vi "Data Folder.vi"(8 "error in (no error)":errorcluster, 11 "Node Ptr":T2 format="%.0x") -> (0 "error out":errorcluster)   [LabVIEW 2020, in "RefMem DMA System Explorer.lvlib"]
uses:
  RefMem DMA System Explorer.lvlib
  <vilib>/NI VeriStand/Custom Device API/Custom Device Item Ref.ctl
  controls/Data Channel Type.ctl
  <vilib>/NI VeriStand/Custom Device API/Custom Device Channel.ctl
  <vilib>/NI VeriStand/Custom Device API/Custom Device Channel Type.ctl
  Shared/Constants.vi
  <vilib>/NI VeriStand/Custom Device API/Get Item Property (U16).vi
  <vilib>/NI VeriStand/Custom Device API/Get Item Property (U32).vi
  <vilib>/NI VeriStand/Custom Device Tools/Custom Device Utility Library/NI VeriStand - Search for Item by Name.vi
  <vilib>/NI VeriStand/Custom Device API/NI VeriStand - Find next valid Label.vi
  <vilib>/NI VeriStand/Custom Device API/Set Item Property (U16).vi
  <vilib>/NI VeriStand/Custom Device API/Set Item Property (U32).vi
  <vilib>/NI VeriStand/Custom Device API/Custom Device API.lvlib
  Shared/RefMem DMA Shared.lvlib
  <vilib>/NI VeriStand/Custom Device Tools/Custom Device Utility Library/Custom Device Utility Library.lvlib
panel:
  in  "Type":T1
  in  "Block Address":u32
  in  "Add Data Channel":bool
  in  "Header":cluster{"Section Name":string}={"Section Name"="Data Folder"}
  in  "Description":string
  in  "Name":string
  # "In channels (doubles)"
  # "Channels to write has to be in row\nChannels to read can have space in between"
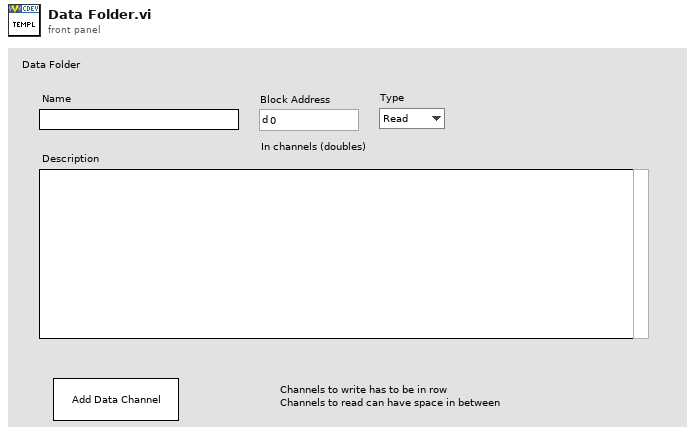
[diagram p1: front panel]
types:
  T1 = typedef "RefMem DMA System Explorer.lvlib/Data Channel Type.ctl" = enum16{"Read", "Write"}
  T2 = typedef "Custom Device API.lvlib/Custom Device Item Ref.ctl" = u64
  T3 = typedef "Custom Device API.lvlib/Custom Device Item Info.ctl" = cluster{"Name":string, "Is Channel":bool, "GUID":string, "Is Waveform":bool}
  T4 = typedef "Custom Device API.lvlib/Custom Device Channel.ctl" = cluster{"Type":T5, "Units":string, "Default Value":dbl, "Faultable":bool, "Scalable":bool}
  T5 = typedef "Custom Device API.lvlib/Custom Device Channel Type.ctl" = enum16{"Input", "Output"}
  T6 = typedef "Custom Device API.lvlib/Custom Device Commands.ctl" = enum16{"Default", "Item renamed", "Shutdown", "Dynamic button pressed"}
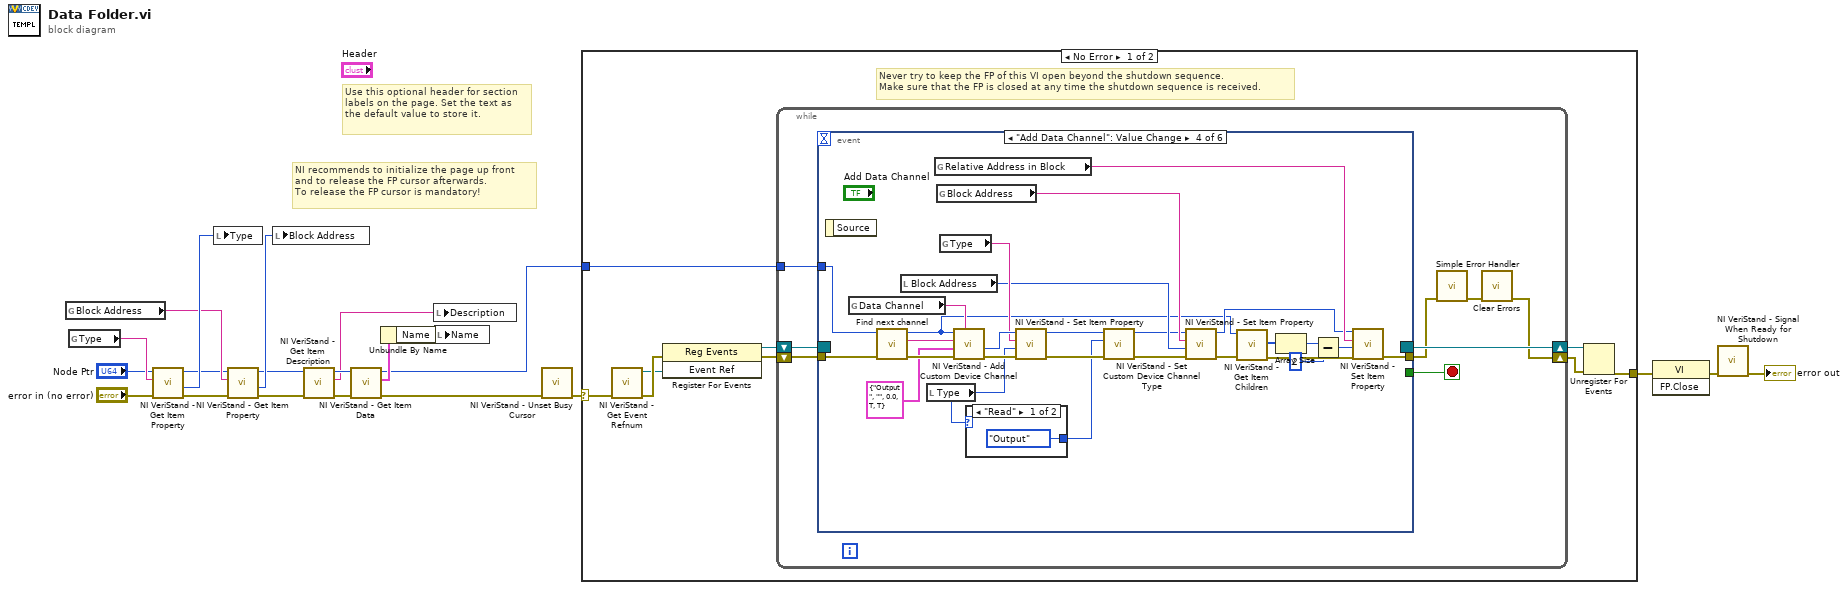
[diagram p0: block diagram]
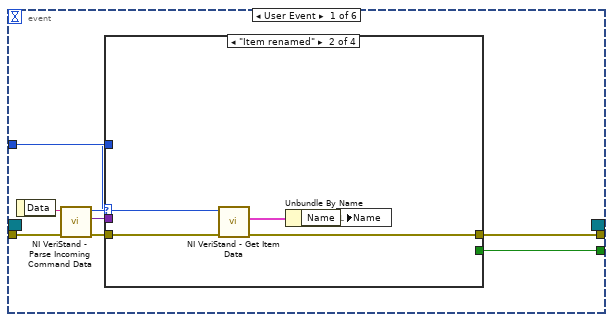
[diagram p2: hidden frame]
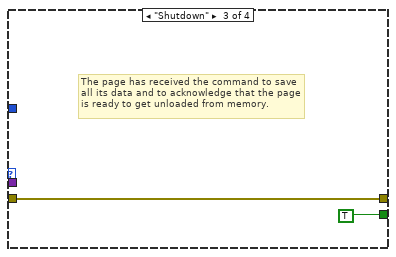
[diagram p4: hidden frame]
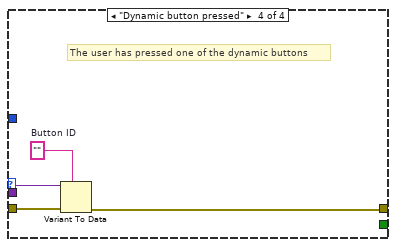
[diagram p5: hidden frame]
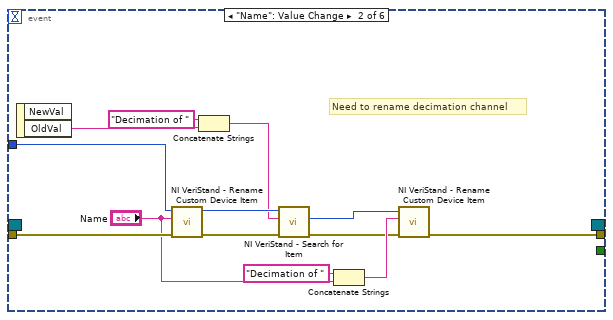
[diagram p6: hidden frame]
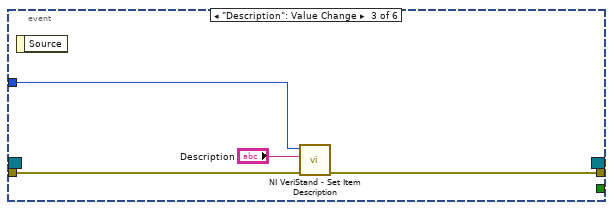
[diagram p7: hidden frame]
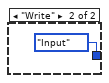
[diagram p8: hidden frame]
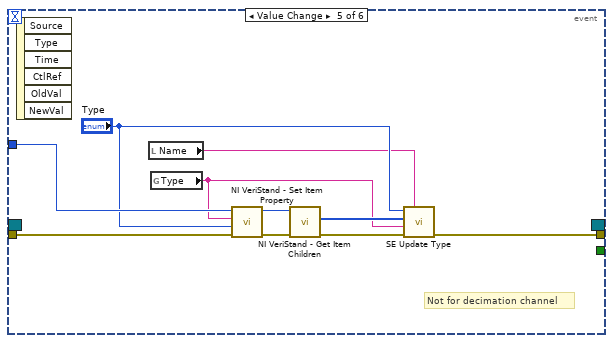
[diagram p9: hidden frame]
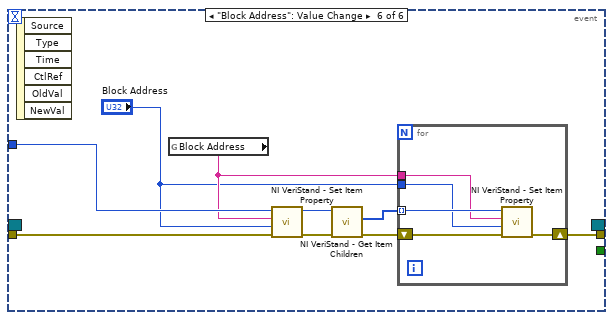
[diagram p10: hidden frame]
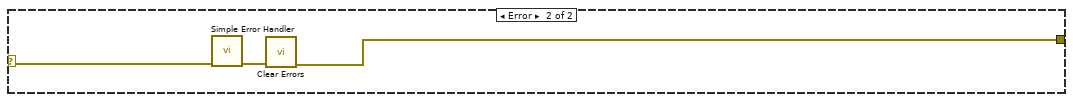
[diagram p11: hidden frame]
diagram:
  # "Use this optional header for section labels on the page. Set the text as the default value to store it."
  # "NI recommends to initialize the page up front\nand to release the FP cursor afterwards.\nTo release the FP cursor is mandatory!"
  n1 = global read "Constants.vi" "Block Address"() -> (w9:string)
  n2 = global read "Constants.vi" "Type"() -> (w12:string)
  n3 = call-poly <vilib>:"NI VeriStand - Get Item Property.vi"("error in (no error)"="error in (no error)", "Property Name"=w12, "Item Ref in"="Node Ptr") -> ("error out"=w5:errorcluster, "Value"=w11:u16, "Item Ref out"=w4:T2)  [unwired: 5 in, 1 out]
  n4 = local write "Type"(w11) -> ()
  n5 = call-poly <vilib>:"NI VeriStand - Get Item Property.vi"("error in (no error)"=w5, "Property Name"=w9, "Item Ref in"=w4) -> ("error out"=w1:errorcluster, "Value"=w10:u32, "Item Ref out"=w2:T2)  [unwired: 5 in, 1 out]
  n6 = local write "Block Address"(w10) -> ()
  n7 = call <vilib>:"NI VeriStand - Get Item Description.vi"("error in (no error)"=w1, "Item Ref in"=w2) -> ("error out"=w15:errorcluster, "Description"=w16:string, "Item Ref out"=w17:T2)  [unwired: 7 out]
  n8 = call <vilib>:"NI VeriStand - Get Item Data.vi"("error in (no error)"=w15, "Item Ref in"=w17) -> ("error out"=w8:errorcluster, "Item Info"=w14:T3, "Item Ref out"=w3:T2)  [unwired: 7 out]
  n9 = Unbundle By Name(w14) -> ("Name"=w13:string)
  n10 = local write "Description"(w16) -> ()
  n11 = local write "Name"(w13) -> ()
  n12 = call <vilib>:"NI VeriStand - Unset Busy Cursor.vi"("error in (no error)"=w8) -> ("error out"=w18:errorcluster)  [unwired: 10 out]
  n13 = case shown="No Error" w18 {
    selector: w18 -> [w22 w131]
    tunnel: [w27 w129] -> w21
    tunnel: w3 -> [w23 _]
    frame No Error {
      # "Never try to keep the FP of this VI open beyond the shutdown sequence.\nMake sure that the FP is closed at any time the shutdown sequence is received."
      n14 = call <vilib>:"NI VeriStand - Get Event Refnum.vi"("error in (no error)"=w22) -> ("error out"=w30:errorcluster, "Event Ref"=w26:refnum<user-event>)  [unwired: 9 out]
      n15 = register-events(error in=w30, w26) -> (reference out=w24:refnum<event-registration>, error out=w25:errorcluster)  [unwired: 1 in]
      n16 = while {
        tunnel: w23 -> [w34]
        shift-right: [w31] -> w28
        shift-left: w25 -> [w37]
        shift-right: [w38] -> w29
        shift-left: w24 -> [w36]
        stop <- w35 stop-if-true
        n17 = event shown="[3] \"Add Data Channel\": Value Change" {
          selector: w36 -> [_ _ _ _ _ _]
          dyn-events: [_ _ _ _ _ _] -> w38
          timeout: _ -> [_ _ _ _ _ _]
          tunnel: w37 -> [w46 w71 w74 w101 w114 w123]
          tunnel: [w42 _ _ _ _ _] -> w35
          tunnel: [w41 w66 w73 w91 w113 w118] -> w33
          tunnel: w34 -> [w40 w70 w75 w100 w112 w122]
          event User Event {
            n18 = event-data() -> ("Data"=w45:string)  [unwired: 1 out]
            n19 = call <vilib>:"NI VeriStand - Parse Incoming Command Data.vi"("error in (no error)"=w46, "Incoming data"=w45) -> ("error out"=w44:errorcluster, "Outgoing data"=w39:variant, "Action"=w43:T6)  [unwired: 7 out]
            n20 = case shown="\"Item renamed\"" w43 {
              tunnel: w44 -> [w47 w52 w53 w58]
              tunnel: [_ _ TRUE _] -> w42
              tunnel: [w47 w49 w53 w55] -> w41
              tunnel: w40 -> [_ w51 _ _]
              tunnel: w39 -> [_ _ _ w57]
              frame "Default", Default {
              }
              frame "Item renamed" {
                n21 = call <vilib>:"NI VeriStand - Get Item Data.vi"("error in (no error)"=w52, "Item Ref in"=w51) -> ("error out"=w49:errorcluster, "Item Info"=w50:T3)  [unwired: 8 out]
                n22 = Unbundle By Name(w50) -> ("Name"=w48:string)
                n23 = local write "Name"(w48) -> ()
              }
              frame "Shutdown" {
                # "The page has received the command to save all its data and to acknowledge that the page is ready to get unloaded from memory."
              }
              frame "Dynamic button pressed" {
                w56 = ""  # Button ID
                # "The user has pressed one of the dynamic buttons"
                n24 = Variant To Data(error in=w58, type=w56, Variant=w57) -> (error out=w55:errorcluster)  [unwired: 1 out]
              }
            }
          }
          event "Name": Value Change {
            # "Need to rename decimation channel"
            n25 = event-data() -> ("OldVal"=w60:string)  [unwired: 2 out]
            n26 = call <vilib>:"NI VeriStand - Rename Custom Device Item.vi"("error in (no error)"=w71, "New Name"="Name", "Item Ref in"=w70) -> ("error out"=w64:errorcluster, "Item Ref out"=w65:T2)  [unwired: 1 in, 6 out]
            n27 = Concatenate Strings("Decimation of " ("string"), w60) -> (w59:string)
            n28 = call-poly <vilib>:"NI VeriStand - Search for Item.vi"("error in"=w64, "Item Name"=w59, "Section Ref in"=w65) -> ("error out"=w63:errorcluster, "Item Ref"=w62:T2)  [unwired: 5 in, 2 out]
            n29 = Concatenate Strings("Decimation of " ("string"), "Name") -> (w67:string)
            n30 = call <vilib>:"NI VeriStand - Rename Custom Device Item.vi"("error in (no error)"=w63, "New Name"=w67, "Item Ref in"=w62) -> ("error out"=w66:errorcluster)  [unwired: 1 in, 7 out]
          }
          event "Description": Value Change {
            n31 = event-data() -> ()  [unwired: 2 out]
            n32 = call <vilib>:"NI VeriStand - Set Item Description.vi"("error in (no error)"=w74, "Description"="Description", "Item Ref in"=w75) -> ("error out"=w73:errorcluster)  [unwired: 8 out]
          }
          event "Add Data Channel": Value Change {
            n33 = event-data() -> ()  [unwired: 2 out]
            n34 = global read "Constants.vi" "Data Channel"() -> (w102:string)
            n35 = call "Find next channel.vi"("error in (no error)"=w101, "Item Ref out in"=w100) -> ("error out"=w98:errorcluster, "Label out"=w99:string, "Item Ref out out"=w85:T2)  [unwired: 7 in]
            n36 = local read "Block Address"() -> (w90:u32)
            n37 = local read "Type"() -> (w81:T1)
            n38 = global read "Constants.vi" "Relative Address in Block"() -> (w92:string)
            n39 = global read "Constants.vi" "Block Address"() -> (w93:string)
            n40 = global read "Constants.vi" "Type"() -> (w94:string)
            n41 = call <vilib>:"NI VeriStand - Add Custom Device Channel.vi"("GUID (Default Channel)"=w102, "error in (no error)"=w98, "Channel"=T4 {"Type"=enum."Output", "Units"="", "Default Value"=0.0, "Faultable"=TRUE, "Scalable"=TRUE}, "Channel Name"=w99, "Parent Ref in"=w85) -> ("error out"=w96:errorcluster, "Channel Ref"=w95:T2)  [unwired: 3 in, 2 out]
            n42 = case shown="\"Read\"" w81 {
              tunnel: [Custom_Device_Channel_Type."Output" ("Type") Custom_Device_Channel_Type."Input" ("Type")] -> w78
              frame "Read" {
              }
              frame "Write" {
              }
            }
            n43 = call-poly <vilib>:"NI VeriStand - Set Item Property.vi"("error in (no error)"=w96, "Value"=w81, "Property Name"=w94, "Item Ref in"=w95) -> ("error out"=w79:errorcluster, "Item Ref out"=w80:T2)  [unwired: 5 in, 1 out]
            n44 = call <vilib>:"NI VeriStand - Set Custom Device Channel Type.vi"("error in (no error)"=w79, "Type"=w78, "Channel Ref in"=w80) -> ("error out"=w76:errorcluster, "Channel Ref out"=w77:T2)  [unwired: 7 in]
            n45 = call-poly <vilib>:"NI VeriStand - Set Item Property.vi"("error in (no error)"=w76, "Value"=w90, "Property Name"=w93, "Item Ref in"=w77) -> ("error out"=w89:errorcluster, "Item Ref out"=w86:T2)  [unwired: 5 in, 1 out]
            n46 = call <vilib>:"NI VeriStand - Get Item Children.vi"("error in (no error)"=w89, "Item Ref in"=w85) -> ("error out"=w88:errorcluster, "Child Refs"=w87:T2[])  [unwired: 6 in, 2 out]
            n47 = Array Size(array=w87) -> (size(s)=w84:i32)
            n48 = Subtract(x=w84, y=2) -> (x-y=w83:i32)
            n49 = call-poly <vilib>:"NI VeriStand - Set Item Property.vi"("error in (no error)"=w88, "Value"=w83, "Property Name"=w92, "Item Ref in"=w86) -> ("error out"=w91:errorcluster)  [unwired: 5 in, 2 out]
          }
          event Value Change {
            # "Not for decimation channel"
            n50 = event-data() -> ()  [unwired: 7 out]
            n51 = local read "Name"() -> (w107:string)
            n52 = global read "Constants.vi" "Type"() -> (w105:string)
            n53 = call-poly <vilib>:"NI VeriStand - Set Item Property.vi"("error in (no error)"=w114, "Value"="Type", "Property Name"=w105, "Item Ref in"=w112) -> ("error out"=w110:errorcluster, "Item Ref out"=w111:T2)  [unwired: 5 in, 1 out]
            n54 = call <vilib>:"NI VeriStand - Get Item Children.vi"("error in (no error)"=w110, "Item Ref in"=w111) -> ("error out"=w109:errorcluster, "Child Refs"=w106:T2[])  [unwired: 6 in, 2 out]
            n55 = call "SE Update Type.vi"("Name"=w107, "error in (no error)"=w109, 9:"Type"=w105, "Child Refs"=w106, 11:"Type"="Type") -> ("error out"=w113:errorcluster)  [unwired: 6 in]
          }
          event "Block Address": Value Change {
            n56 = event-data() -> ()  [unwired: 7 out]
            n57 = global read "Constants.vi" "Block Address"() -> (w117:string)
            n58 = call-poly <vilib>:"NI VeriStand - Set Item Property.vi"("error in (no error)"=w123, "Value"="Block Address", "Property Name"=w117, "Item Ref in"=w122) -> ("error out"=w121:errorcluster, "Item Ref out"=w120:T2)  [unwired: 5 in, 1 out]
            n59 = call <vilib>:"NI VeriStand - Get Item Children.vi"("error in (no error)"=w121, "Item Ref in"=w120) -> ("error out"=w119:errorcluster, "Child Refs"=w116:T2[])  [unwired: 6 in, 2 out]
            n60 = for {
              shift-right: [w127] -> w118
              shift-left: w119 -> [w128]
              tunnel: w117 -> [w125]
              tunnel: w116 -> [w126] mode=indexing
              tunnel: "Block Address" -> [w124]
              n61 = call-poly <vilib>:"NI VeriStand - Set Item Property.vi"("error in (no error)"=w128, "Value"=w124, "Property Name"=w125, "Item Ref in"=w126) -> ("error out"=w127:errorcluster)  [unwired: 5 in, 2 out]
            }
          }
        }
        n62 = call <vilib>:"Simple Error Handler.vi"("error in (no error)"=w33) -> ("error out"=w32:errorcluster)  [unwired: 1 in, 7 out]
        n63 = call <vilib>:"Clear Errors.vi"("error in (no error)"=w32) -> ("error out"=w31:errorcluster)  [unwired: 1 in, 5 out]
      }
      n64 = Unregister For Events(event registration refnum=w29, error in=w28) -> (error out=w27:errorcluster)
    }
    frame Error {
      n65 = call <vilib>:"Simple Error Handler.vi"("error in (no error)"=w131) -> ("error out"=w130:errorcluster)  [unwired: 1 in, 7 out]
      n66 = call <vilib>:"Clear Errors.vi"("error in (no error)"=w130) -> ("error out"=w129:errorcluster)  [unwired: 1 in, 5 out]
    }
  }
  n67 = invoke class="VI" method="FP.Close"(error in=w21) -> (error out=w20:errorcluster)  [unwired: 2 in, 2 out]
  n68 = call <vilib>:"NI VeriStand - Signal When Ready for Shutdown.vi"("error in (no error)"=w20) -> ("error out"=→"error out":errorcluster)  [unwired: 10 out]
